vi "InHouseJSONParser.vi"(8 "error in (no error)":errorcluster, 11 "feGEM JSON string":string) -> (0 "error out":errorcluster, 2 "Settings file as array":string[](array[string]), 3 "JSON as array":string[](array[string]))   [LabVIEW 2018]
panel:
  out "JSON with no witespace":string
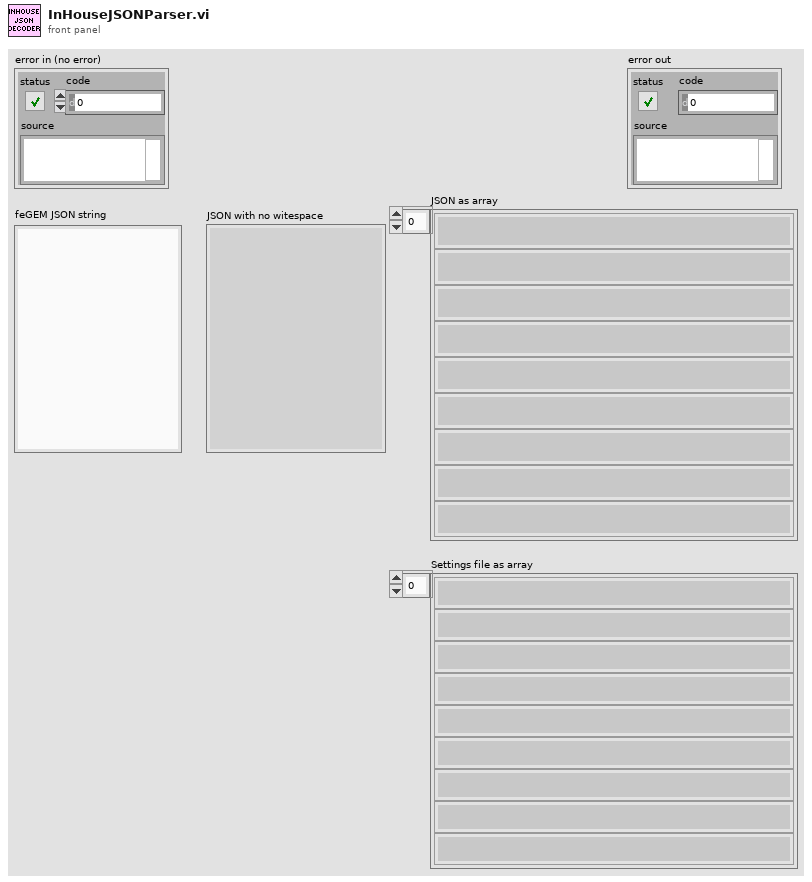
[diagram p1: front panel]
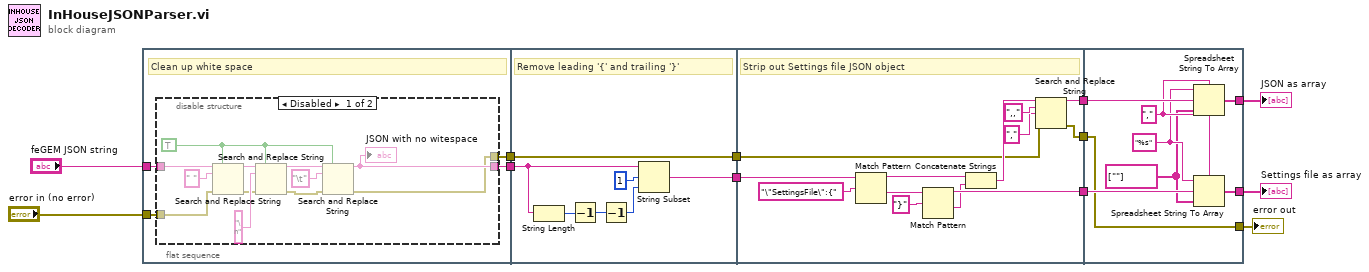
[diagram p0: block diagram]
diagram:
  n1 = flat-sequence {
    tunnel: "feGEM JSON string" -> [w16]
    tunnel: [w15] -> w11
    tunnel: "error in (no error)" -> [w14]
    tunnel: [w13] -> w3
    tunnel: w11 -> [w36]
    tunnel: [w32] -> w10
    tunnel: [w31] -> w4
    tunnel: w3 -> [w31]
    tunnel: w10 -> [w49]
    tunnel: [w45] -> w9
    tunnel: [w40] -> w8
    tunnel: w4 -> [w39]
    tunnel: [w38] -> w2
    tunnel: w9 -> [w54]
    tunnel: w8 -> [w58]
    tunnel: [w57] -> w7
    tunnel: [w52] -> w6
    tunnel: w2 -> [w51]
    tunnel: [w51] -> w1
    frame #0 {
      # "Clean up white space"
      n2 = disable-structure shown="Disabled" {
        disable-tunnel: w16 -> [w28 w30]
        disable-tunnel: [w22 w30] -> w15
        disable-tunnel: w14 -> [w20 w29]
        disable-tunnel: [w17 w29] -> w13
        frame Disabled {
          w21 = TRUE ("replace all? (F)")
          n3 = Search and Replace String(replace all?=w21, input string=w28, search string=" ", error in=w20) -> (result string=w26:string, error out=w19:errorcluster)  [unwired: 4 in, 2 out]
          n4 = Search and Replace String(replace all?=w21, input string=w26, search string="\n", error in=w19) -> (result string=w24:string, error out=w18:errorcluster)  [unwired: 4 in, 2 out]
          n5 = Search and Replace String(replace all?=w21, input string=w24, search string="\t", error in=w18) -> (result string=w22:string, error out=w17:errorcluster)  [unwired: 4 in, 2 out]
          "JSON with no witespace" <- w22
        }
        frame Enabled {
        }
      }
    }
    frame #1 {
      # "Remove leading '{' and trailing '}'"
      n6 = String Length(string=w36) -> (length=w35:i32)
      n7 = Decrement(x=w35) -> (x-1=w34:i32)
      n8 = Decrement(x=w34) -> (x-1=w33:i32)
      n9 = String Subset(string=w36, offset (0)=1, length (rest)=w33) -> (substring=w32:string)
    }
    frame #2 {
      # "Strip out Settings file JSON object"
      n10 = Match Pattern(string=w49, regular expression="\"SettingsFile\":{") -> (before substring=w48:string, after substring=w47:string)  [unwired: 1 in, 2 out]
      n11 = Match Pattern(string=w47, regular expression="}") -> (before substring=w45:string, after substring=w44:string)  [unwired: 1 in, 2 out]
      n12 = Concatenate Strings(w48, w44) -> (w43:string)
      n13 = Search and Replace String(input string=w43, search string=",,", replace string="," ("replace string (\"\")"), error in=w39) -> (result string=w40:string, error out=w38:errorcluster)  [unwired: 4 in, 2 out]
    }
    frame #3 {
      w55 = "%s" ("format string")
      w56 = "," ("delimiter (Tab)")
      w53 = string[] [""] ("delimiters (\\s,\\t,\\r,\\n)")
      n14 = Spreadsheet String To Array(delimiter (Tab)=w56, format string=w55, spreadsheet string=w58, array type (2D Dbl)=w53) -> (array=w57:string[])
      n15 = Spreadsheet String To Array(delimiter (Tab)=w56, format string=w55, spreadsheet string=w54, array type (2D Dbl)=w53) -> (array=w52:string[])
    }
  }
  "JSON as array" <- w7
  "Settings file as array" <- w6
  "error out" <- w1
